vi "DAQInputVUmeter.vi"() -> ()   [LabVIEW 2015]
panel:
  in  "stop":bool
  out "Data":dbl
  out "Waveform Chart":dynamicdata(graph)
  # "EE2073\nGROUP 1"
  # "ALBERT SOERJONOTO"
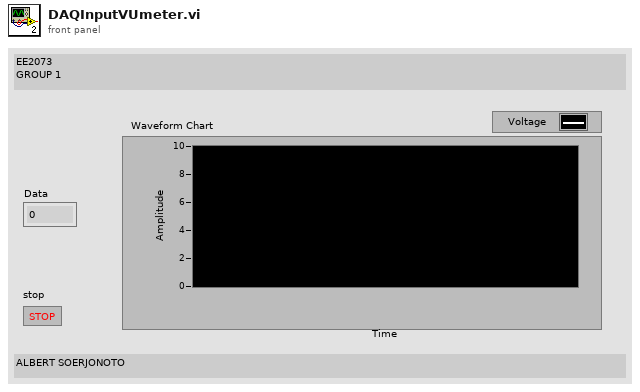
[diagram p1: front panel]
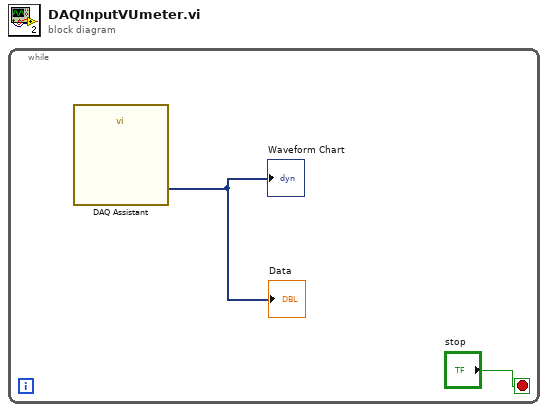
[diagram p0: block diagram]
diagram:
  n1 = while {
    stop <- "stop" stop-if-true
    n2 = call "DAQ Assistant"() -> ("data"=→"Waveform Chart" →"Data":dynamicdata)  [unwired: 16 in, 3 out]
  }
